vi "tcplink publish -- map.vi"(7 "publisher action":T2, 11 "sparkle map IN":map{string, T1}(c390)) -> (3 "sparkle map OUT":map{string, T1}(c390))   [LabVIEW 2020]
uses:
  publisher action.ctl
  sparkle.ctl
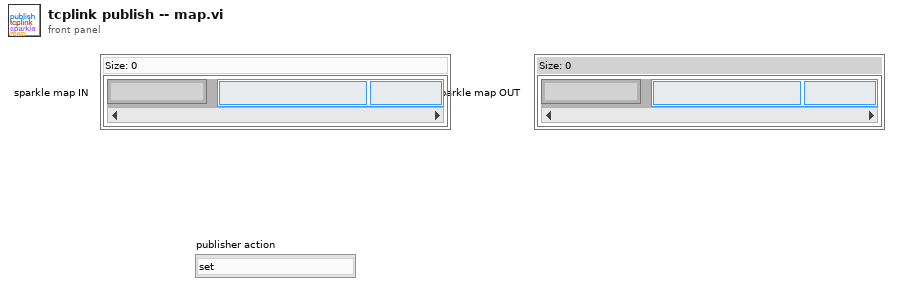
[diagram p1: front panel]
types:
  T1 = typedef "sparkle.ctl" = cluster{"units":string, "data":dbl}
  T2 = typedef "publisher action.ctl" = enum16{"set", "get", "init", "check"}
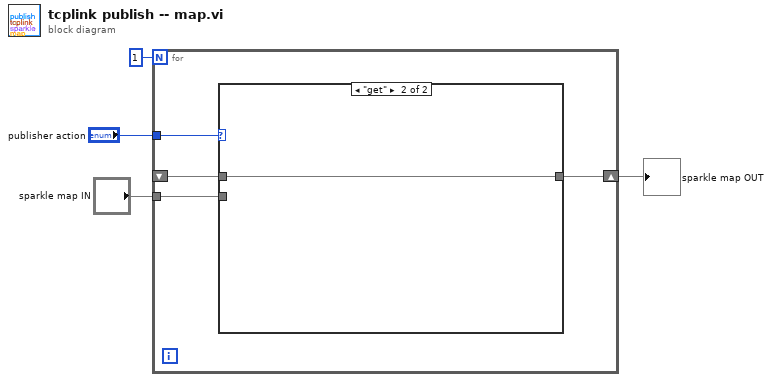
[diagram p0: block diagram]
diagram:
  n1 = for {
    N: 1 -> [_]
    tunnel: "publisher action" -> [w8]
    tunnel: "sparkle map IN" -> [w6]
    shift-right: [w7] -> w2
    shift-left: _ -> [w5]
    n2 = case shown="\"get\"" w8 {
      tunnel: [w9 w10] -> w7
      tunnel: w6 -> [w9 _]
      tunnel: w5 -> [_ w10]
      frame "set", Default {
      }
      frame "get" {
      }
    }
  }
  "sparkle map OUT" <- w2
